vi "Revoke Window Always on Top.vi"(8 "error in":errorcluster caption="error in (no error)" {"code" format="%d\n%x"}, 9 "activate? (F)":bool, 10 "window name (\"\")":string, 11 "window refnum":T1 caption="window refnum (NaWR)") -> (0 "error out":errorcluster {"code" format="%d\n%x"}, 3 "window refnum out":T1)   [LabVIEW 2020, in "Win Util New.lvlib"]
doc: "This function will revoke the topmost status of the window named in the 'window name' input, or identified by the 'window refnum' the topmost window, so it will no longer always be on top of other 'normal' windows. The action is ignored if the window is not a topmost window. If 'not a window refnum' is passed in, then the function will use the window name to get a window window refnum. If the window cannot be found, an error will be returned."
uses:
  Win Util New.lvlib
  Window Refnum.ctl
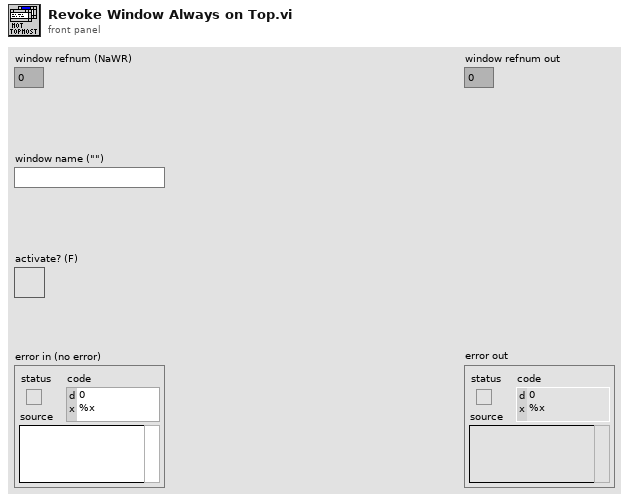
[diagram p1: front panel]
types:
  T1 = typedef "Win Util New.lvlib/Window Refnum.ctl" = u64
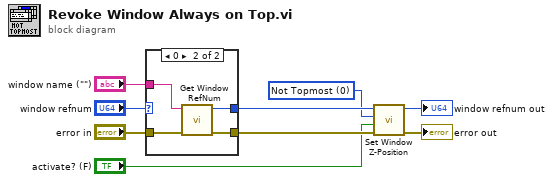
[diagram p0: block diagram]
diagram:
  w4 = u16 0 items=["Not Topmost", "Topmost", "Top", "Bottom"]
  n1 = case shown="0" "window refnum" {
    selector: "window refnum" -> [w10 _]
    tunnel: "error in" -> [w11 w15]
    tunnel: [w10 w14] -> w8
    tunnel: [w11 w13] -> w7
    tunnel: "window name (\"\")" -> [_ w12]
    frame Default {
    }
    frame 0 {
      n2 = call "Get Window RefNum.vi"("error in"=w15, "window name (\"\")"=w12) -> ("error out"=w13:errorcluster, "window refnum (NaWR)"=w14:T1)  [unwired: 6 out]
    }
  }
  n3 = call "Set Window Z-Position.vi"("error in"=w7, "No Activate? (T)"="activate? (F)", "z-order position"=w4, "window refnum"=w8) -> ("error out"=→"error out":errorcluster, "window refnum out"=→"window refnum out":T1)  [unwired: 6 in]
